vi "Creators Creator Queue Alias.vi"(11 "Base Event jettl in":refnum<class "Base Event jettl.lvclass">) -> (2 "Creator Queue Alias":string, 3 "Base Event jettl out":refnum<class "Base Event jettl.lvclass">)   [LabVIEW 2021, in "jettl.lvlib" / "Base Event jettl.lvlib" / "Base Event jettl.lvclass"]
uses:
  Base Event jettl.lvclass
  Base Event jettl.lvclass/Base Event jettl.ctl
  Queue Mailbox/Queue Mailbox.lvlib
  C:/git/jettl/src/jettl/jettl/jettl.lvclass
  C:/git/jettl/src/jettl Msg Merge Error/Merge Error/Merge Error.lvclass
  C:/git/jettl/src/jettl/Event jettl/Event jettl.lvclass
  C:/git/jettl/src/jettl Msg Override Error/Override Error/Override Error.lvclass
  C:/git/jettl/src/jettl Msg Setup/Setup/Setup.lvclass
  C:/git/jettl/src/jettl Msg Teardown/Teardown/Teardown.lvclass
  C:/git/jettl/src/jettl/Base Event jettl/Base Event jettl/Base Event jettl.lvclass
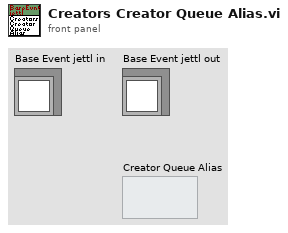
[diagram p1: front panel]
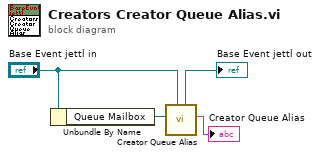
[diagram p0: block diagram]
diagram:
  n1 = Unbundle By Name("Base Event jettl in") -> ("Queue Mailbox"=w4:refnum<data-value>)
  n2 = call "Creator Queue Alias.vi"("jettl in"="Base Event jettl in", "Queue Mailbox"=w4) -> ("Creator Queue Alias"=→"Creator Queue Alias":string, "jettl out"=→"Base Event jettl out":refnum<class "Base Event jettl.lvclass">)  [unwired: 8 in]
